vi "Configure Modulation (Amplitude).vi"(0 "VISA resource name":refnum<visa-resource-name>, 1 "AM Source (0: Internal)":i32(ring) items=["Internal", "External", "CH1", "CH2"], 2 "Modulation Function (0: Sine)":i32(ring) items=["Sine", "Square", "Ramp", "NRamp", "Triangle", "Noise", "PRBS", "ARB"], 5 "Channel (1: 1)":i32(ring)=1 items=["1"=1, "2"=2], 7 "Enable AM (T: Enable)":bool=TRUE, 9 "Enable DSSC (F: Disable)":bool, 11 "error in (no error)":errorcluster, 12 "Modulation Depth (100 Percent)":dbl=100.0, 13 "Modulation Frequency (100 Hz)":dbl=100.0, 14 "Sample Rate (40000 Sa/s)":dbl=40000.0) -> (4 "VISA resource name out":refnum<visa-resource-name>, 15 "error out":errorcluster)   [LabVIEW 2016, in "Agilent 3352X Series.lvlib"]
doc: "Configures and enables amplitude modulation (AM). In AM, the amplitude of the carrier is varied by the amplitude of the modulating waveform. \n\n<B>Note</B>:\n(1) When enabling this mode, all other modes will be turned off.\n(2) The carrier waveform shape and parameters are set by the Configure Standard Waveform VI, Configure PRBS Waveform VI, or Configure Pulse Waveform VI.\n(3) You can Apply any carrier waveform but DC."
uses:
  Agilent 3352X Series.lvlib
panel:
  # "Internal AM Settings"
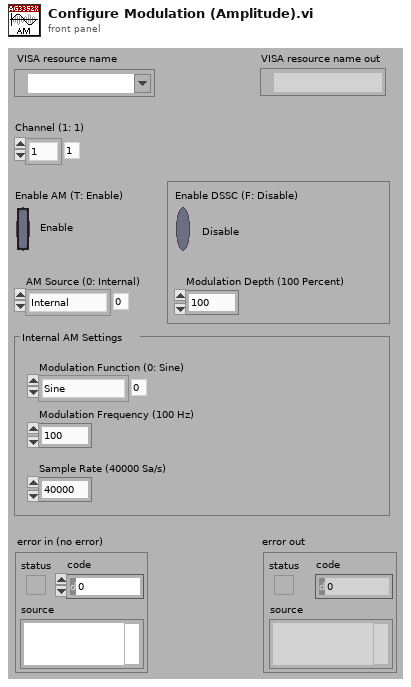
[diagram p1: front panel]
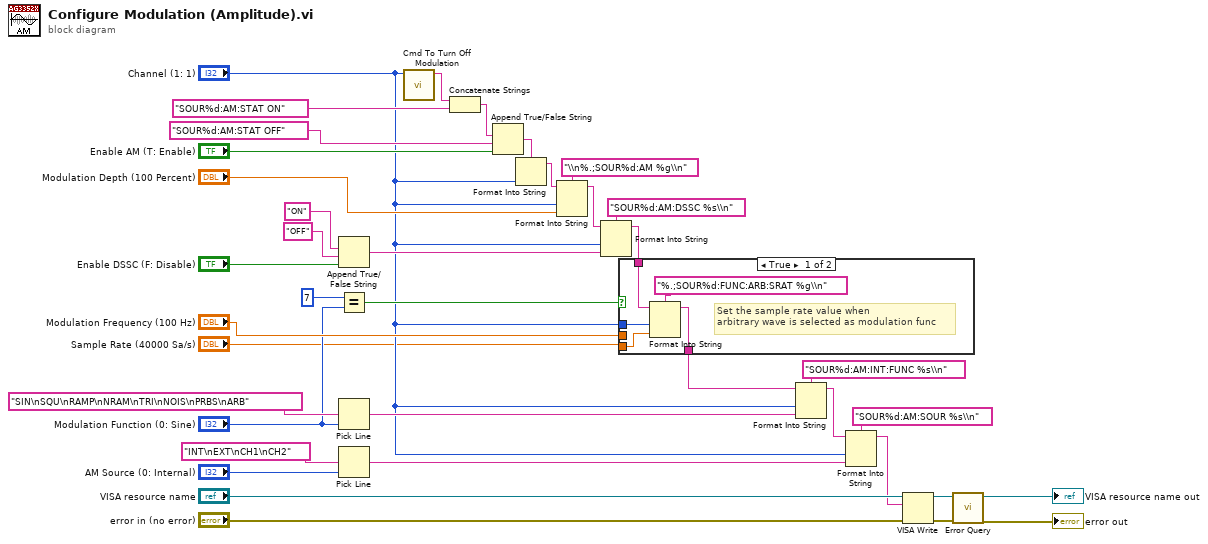
[diagram p0: block diagram]
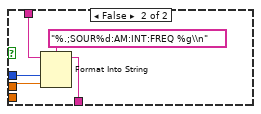
[diagram p2: hidden frame]
diagram:
  n1 = Append True/False String(1:"Enable DSSC (F: Disable)", 2:"OFF", 3:"ON") -> (0:w31:string)  [unwired: 1 out]
  n2 = Equal?(x=u16 7 ("y"), y="Modulation Function (0: Sine)") -> (x = y?=w11:bool)
  n3 = Pick Line(multi-line string="SIN\nSQU\nRAMP\nNRAM\nTRI\nNOIS\nPRBS\nARB", line index="Modulation Function (0: Sine)") -> (output string=w14:string)  [unwired: 1 out]
  n4 = Pick Line(multi-line string="INT\nEXT\nCH1\nCH2", line index="AM Source (0: Internal)") -> (output string=w16:string)  [unwired: 1 out]
  n5 = call "Cmd To Turn Off Modulation.vi"("Channel (1: 1)"="Channel (1: 1)") -> ("Cmd String"=w6:string)  [unwired: 10 out]
  n6 = Concatenate Strings(w6, "SOUR%d:AM:STAT ON") -> (w9:string)
  n7 = Append True/False String(1:"Enable AM (T: Enable)", 2:"SOUR%d:AM:STAT OFF", 3:w9) -> (0:w8:string)  [unwired: 1 out]
  n8 = Format Into String(format string=w8, "Channel (1: 1)") -> (resulting string=w4:string)  [unwired: 2 in, 1 out]
  n9 = Format Into String(format string="\\n%.;SOUR%d:AM %g\\n", initial string=w4, "Channel (1: 1)", "Modulation Depth (100 Percent)") -> (resulting string=w33:string)  [unwired: 1 in, 1 out]
  n10 = Format Into String(format string="SOUR%d:AM:DSSC %s\\n", initial string=w33, "Channel (1: 1)", w31) -> (resulting string=w30:string)  [unwired: 1 in, 1 out]
  n11 = case shown="True" w11 {
    tunnel: "Channel (1: 1)" -> [w41 w48]
    tunnel: w30 -> [w40 w47]
    tunnel: "Modulation Frequency (100 Hz)" -> [_ w45]
    tunnel: [w43 w44] -> w28
    tunnel: "Sample Rate (40000 Sa/s)" -> [w39 _]
    frame True {
      # "Set the sample rate value when\narbitrary wave is selected as modulation func"
      n12 = Format Into String(format string="%.;SOUR%d:FUNC:ARB:SRAT %g\\n", initial string=w40, w41, w39) -> (resulting string=w43:string)  [unwired: 1 in, 1 out]
    }
    frame False {
      n13 = Format Into String(format string="%.;SOUR%d:AM:INT:FREQ %g\\n", initial string=w47, w48, w45) -> (resulting string=w44:string)  [unwired: 1 in, 1 out]
    }
  }
  n14 = Format Into String(format string="SOUR%d:AM:INT:FUNC %s\\n", initial string=w28, "Channel (1: 1)", w14) -> (resulting string=w26:string)  [unwired: 1 in, 1 out]
  n15 = Format Into String(format string="SOUR%d:AM:SOUR %s\\n", initial string=w26, "Channel (1: 1)", w16) -> (resulting string=w10:string)  [unwired: 1 in, 1 out]
  n16 = VISA Write(VISA resource name="VISA resource name", write buffer=w10, error in (no error)="error in (no error)") -> (VISA resource name out=w22:refnum<visa-resource-name>, error out=w21:errorcluster)  [unwired: 1 out]
  n17 = call "Error Query.vi"("error in (no error)"=w21, "VISA resource name"=w22) -> ("error out"=→"error out":errorcluster, "VISA resource name out"=→"VISA resource name out":refnum<visa-resource-name>)  [unwired: 8 out]
